vi "ATMonochromator_getEvent_settingsAppliedMonochromatorRanges.vi"(8 "error in (no error)":errorcluster, 11 "logevent_settingsAppliedMonochromatorRanges_Ctl":T1) -> (0 "error out":errorcluster, 2 "function return":i32, 3 "logevent_settingsAppliedMonochromatorRanges_Ctl out":T1)   [LabVIEW 2016, in "SALLV_ATMonochromator.lvlib"]
doc: "int ATMonochromator_shm_getEvent_settingsAppliedMonochromatorRangesLV(ATMonochromator_logevent_settingsAppliedMonochromatorRangesLV *logevent_settingsAppliedMonochromatorRanges_Ctl );"
uses:
  SALLV_ATMonochromator.lvlib
  DataTypes/logevent_settingsAppliedMonochromatorRanges.ctl
  SALLV_ATMonochromator.so
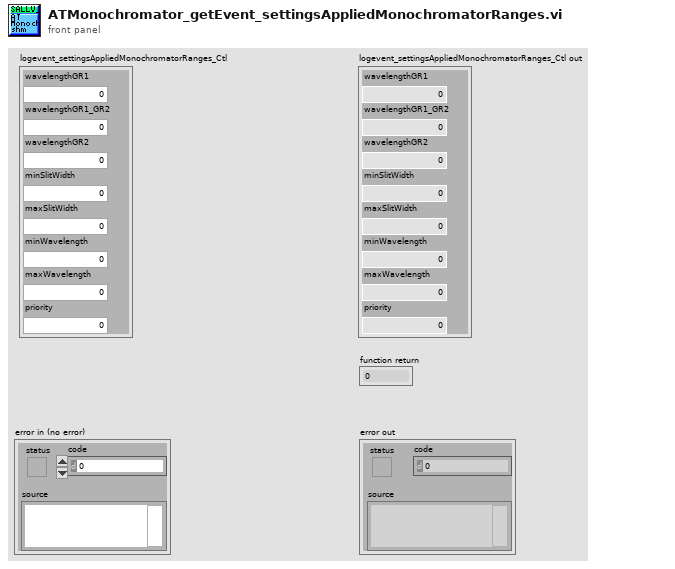
[diagram p1: front panel]
types:
  T1 = typedef "SALLV_ATMonochromator.lvlib/logevent_settingsAppliedMonochromatorRanges.ctl" = cluster{"wavelengthGR1":sgl, "wavelengthGR1_GR2":sgl, "wavelengthGR2":sgl, "minSlitWidth":sgl, "maxSlitWidth":sgl, "minWavelength":sgl, "maxWavelength":sgl, "priority":i32}
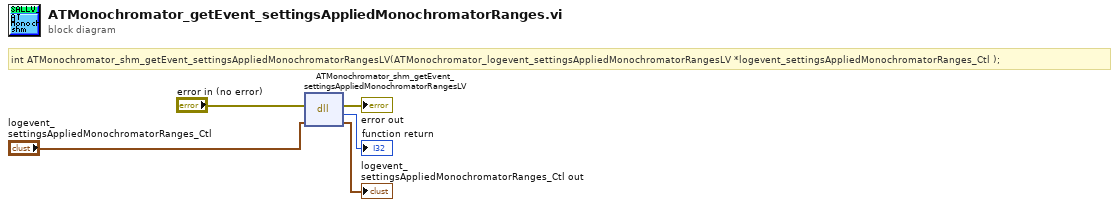
[diagram p0: block diagram]
diagram:
  # "int ATMonochromator_shm_getEvent_settingsAppliedMonochromatorRangesLV(ATMonochromator_logevent_settingsAppliedMonochromatorRangesLV *logevent_settingsAppliedMonochromatorRanges_Ctl );"
  n1 = dll-call lib="home/harini/tcs/SALLV_ATMonochromator/SALLV_ATMonochromator.*" fn="ATMonochromator_shm_getEvent_settingsAppliedMonochromatorRangesLV"(error in="error in (no error)", "logevent_settingsAppliedMonochromatorRanges_Ctl"="logevent_settingsAppliedMonochromatorRanges_Ctl") -> (error out=→"error out":errorcluster, →"function return":i32, "logevent_settingsAppliedMonochromatorRanges_Ctl"=→"logevent_settingsAppliedMonochromatorRanges_Ctl out":T1)  [unwired: 2 in, 1 out]
